vi "StringTo2dFloatArray.vi"(1 "string in":string) -> (0 "Array 2":dbl[][](array[numeric]))   [LabVIEW 2015]
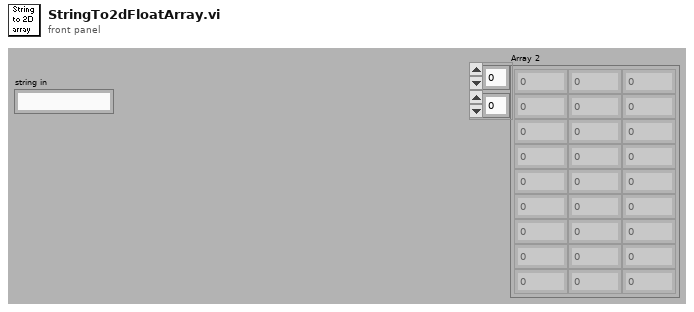
[diagram p1: front panel]
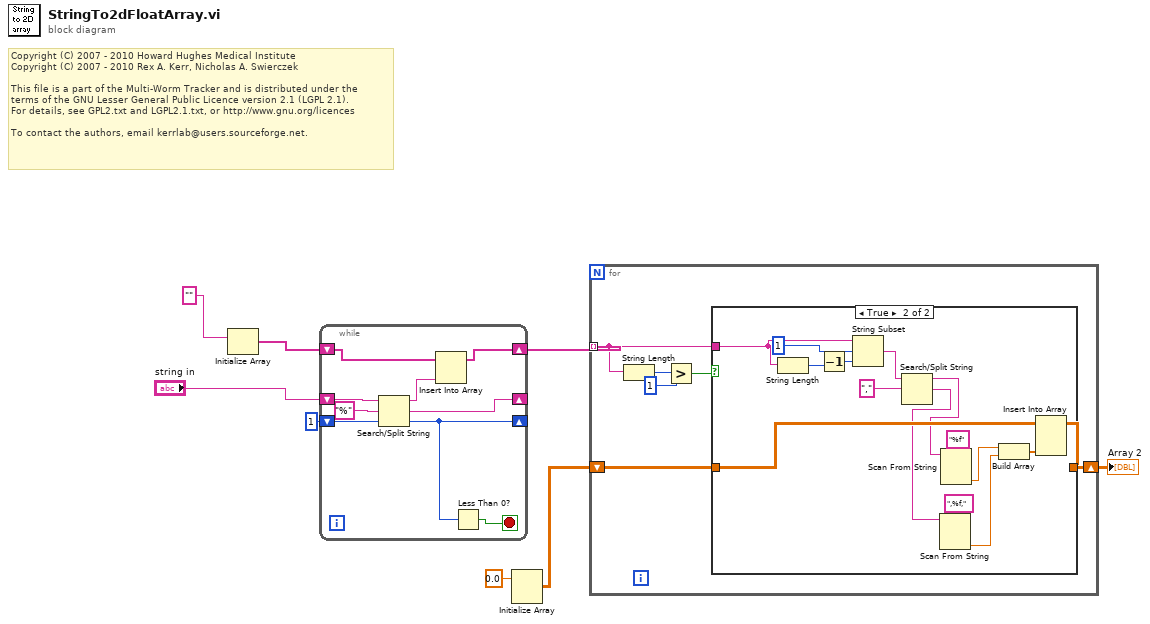
[diagram p0: block diagram]
diagram:
  # "Copyright (C) 2007 - 2010 Howard Hughes Medical Institute\nCopyright (C) 2007 - 2010 Rex A. Kerr, Nicholas A. Swierczek\n \nThis file is a part of the Multi-Worm Tracker and is distributed under the\nterms of the GNU Lesser General Public Licence version 2.1 (LGPL 2.1).\nFor details, see GPL2.txt and LGPL2.1.txt, or http://www.gnu.org/licences\n \nTo contact the authors, email kerrlab@users.sourceforge.net."
  n1 = Initialize Array("") -> (w6:string[])  [unwired: 1 in]
  n2 = while {
    shift-right: [w14] -> _
    shift-left: 1 ("offset of match") -> [w13]
    shift-right: [w12] -> _
    shift-left: "string in" -> [w17]
    shift-right: [w9] -> w4
    shift-left: w6 -> [w11]
    stop <- w16 stop-if-true
    n3 = Search/Split String(string=w17, search string/char (-)="%", offset (0)=w13) -> (substring before match=w10:string, match + rest of string=w12:string, offset of match=w14:i32)
    n4 = Insert Into Array(array=w11, new element=w10) -> (w9:string[])  [unwired: 1 in]
    n5 = Less Than 0?(x=w14) -> (x < 0?=w16:bool)
  }
  n6 = Initialize Array(0.0 ("element")) -> (w3:dbl[][])  [unwired: 2 in]
  n7 = for {
    tunnel: w4 -> [w21] mode=indexing
    shift-right: [w22] -> w1
    shift-left: w3 -> [w23]
    n8 = String Length(string=w21) -> (length=w19:i32)
    n9 = Greater?(x=w19, y=1) -> (0:w20:bool)
    n10 = case shown="True" w20 {
      tunnel: w23 -> [w24 w34]
      tunnel: [w24 w33] -> w22
      tunnel: w21 -> [_ w25]
      frame False {
      }
      frame True {
        n11 = String Length(string=w25) -> (length=w37:i32)
        n12 = Decrement(x=w37) -> (x-1=w36:i32)
        n13 = String Subset(string=w25, offset (0)=1, length (rest)=w36) -> (substring=w35:string)
        n14 = Search/Split String(string=w35, search string/char (-)=",") -> (substring before match=w31:string, match + rest of string=w27:string)  [unwired: 1 in, 1 out]
        n15 = Scan From String(format string=",%f,", input string=w27) -> (output 1=w28:dbl)  [unwired: 3 in, 3 out]
        n16 = Scan From String(format string="%f", input string=w31) -> (output 1=w30:dbl)  [unwired: 3 in, 3 out]
        n17 = Build Array(w30, w28) -> (w32:dbl[])
        n18 = Insert Into Array(array=w34, new element=w32) -> (w33:dbl[][])  [unwired: 2 in]
      }
    }
  }
  "Array 2" <- w1
